vi "Put ECID Data.vi"(8 "error in":errorcluster, 10 "ECID Data":T1, 11 "ECID":u32) -> (0 "error out":errorcluster, 3 "Find?":bool)   [LabVIEW 2020, in "SECS Communication.lvlib" / "SECS Data Class.lvclass"]
uses:
  SECS Data Class.lvclass
  ECID Data.ctl
  SECS-II Class/Format Code.ctl
  SECS-II Class/SECS-II Class.lvclass
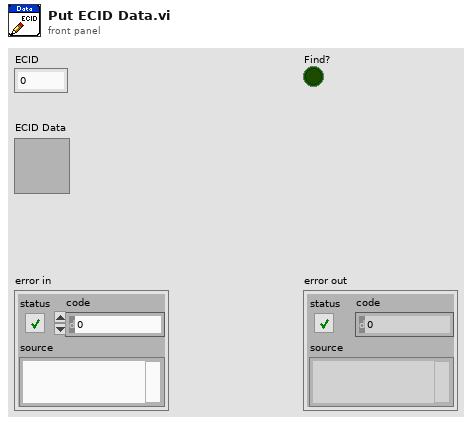
[diagram p1: front panel]
types:
  T1 = typedef "SECS Communication.lvlib/SECS Data Class.lvclass/ECID Data.ctl" = cluster{"ECID":u32, "Name":string, "Description":string, "Format Code":T2, "Unit":string, "Max":dbl, "Min":dbl, "Default":string, "Source":string, "Data":variant}
  T2 = typedef "SECS Communication.lvlib/SECS-II Class.lvclass/Format Code.ctl" = enum16{"L", "A", "B", "Boolean", "J", "I1", "I2", "I4", "I8", "U1", "U2", "U4", "U8", "F4", "F8", "Char"}
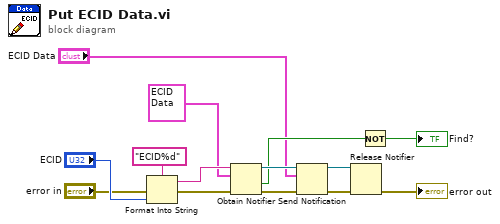
[diagram p0: block diagram]
diagram:
  n1 = Format Into String(format string="ECID%d", error in="error in", "ECID") -> (resulting string=w8:string, error out=w9:errorcluster)  [unwired: 1 in]
  n2 = Obtain Notifier(name (unnamed)=w8, notification data type=T1 {"ECID"=0, "Name"="", "Description"="", "Format Code"=enum."L", "Unit"="", "Max"=0.0, "Min"=0.0, "Default"="", "Source"="", "Data"=variant} ("ECID Data"), error in (no error)=w9) -> (notifier out=w14:refnum<notifier>, created new?=w4:bool, error out=w13:errorcluster)  [unwired: 1 in]
  n3 = Send Notification(notification="ECID Data", notifier=w14, error in (no error)=w13) -> (notifier out=w12:refnum<notifier>, error out=w11:errorcluster)
  n4 = Release Notifier(notifier=w12, error in (no error)=w11) -> (error out=→"error out":errorcluster)  [unwired: 1 in, 2 out]
  n5 = Not(x=w4) -> (.not. x?=→"Find?":bool)
